vi "SNR_SINAD_THD.vi"(8 "error in (no error)":errorcluster caption="错误输入（无错误）", 9 "THD Power Spectrum":cluster{"f0":dbl, "df":dbl, "magnitude":dbl[]}[](array[cluster]), 10 "Harmonics Data Out":dbl[](array[numeric]), 11 "F_Waveform输入":waveform(dbl) caption="F_Waveform输出") -> (0 "error out":errorcluster caption="错误输出", 1 "THD (dB)":dbl, 2 "SNR Power Spectrum":cluster{"f0":dbl, "df":dbl, "magnitude":dbl[]}[](array[cluster]), 3 "SINAD Power Spectrum":cluster{"f0":dbl, "df":dbl, "magnitude":dbl[]}[](array[cluster]), 4 "SINAD (dB)":dbl, 5 "SNR (dB)":dbl)   [LabVIEW 2019]
uses:
  <vilib>/measure/maspectr.llb/FFT Power Spectrum for 1 Chan.vi
  <vilib>/measure/NI_MAPro.lvlib
  <vilib>/Analysis/NI_AALBase.lvlib
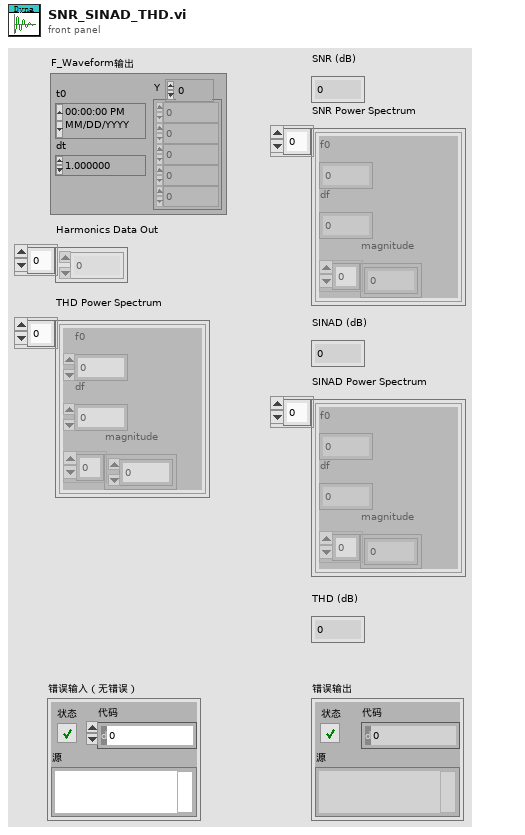
[diagram p1: front panel]
types:
  T1 = enum16{"None ", "Hanning", "Hamming", "Blackman-Harris", "Exact Blackman", "Blackman", "Flat Top", "4 Term B-Harris ", "7 Term B-Harris", "Low Sidelobe"}
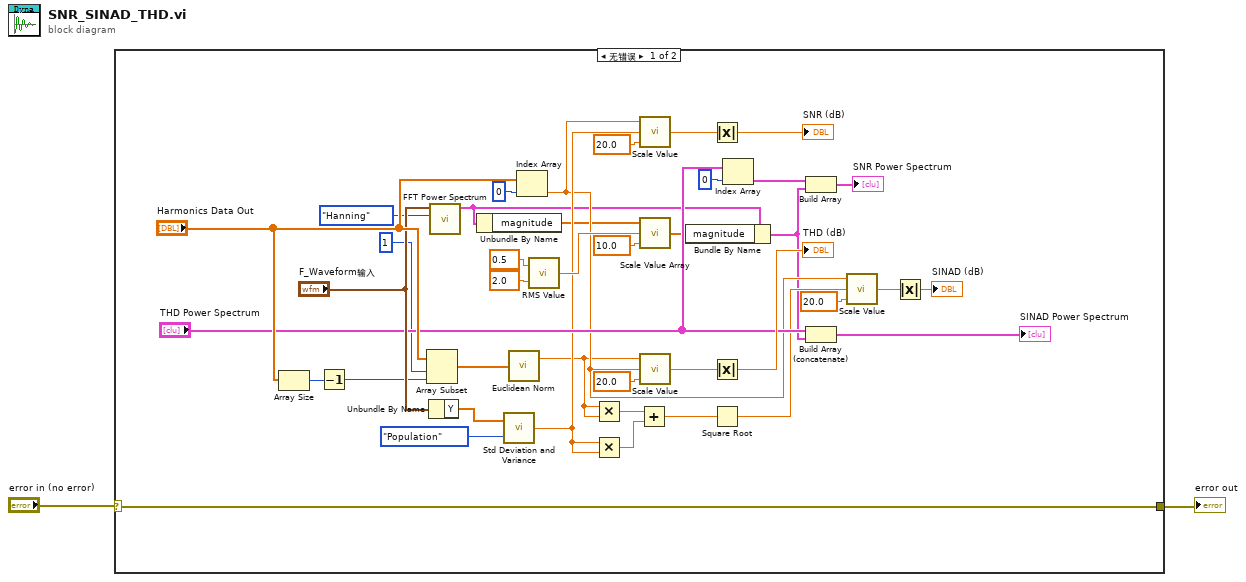
[diagram p0: block diagram]
diagram:
  n1 = case shown="无错误" "error in (no error)" {
    selector: "error in (no error)" -> [w3 w43]
    tunnel: [w3 w43] -> w1
    frame No Error {
      n2 = Array Size(array="Harmonics Data Out") -> (size(s)=w14:i32)
      n3 = Decrement(x=w14) -> (x-1=w13:i32)
      n4 = Array Subset(array="Harmonics Data Out", index=1, length=w13) -> (w10:dbl[])
      n5 = Unbundle By Name("F_Waveform输入") -> ("Y"=w5:dbl[])
      n6 = call-poly <vilib>:"FFT Power Spectrum.vi"("window"=T1."Hanning", "time signal"="F_Waveform输入") -> ("power spectrum"=w23:cluster{"f0":dbl, "df":dbl, "magnitude":dbl[]})  [unwired: 6 in, 3 out]
      n7 = Unbundle By Name(w23) -> ("magnitude"=w20:dbl[])
      n8 = call <vilib>:"Std Deviation and Variance.vi"("X"=w5, "Weighting (Sample)"=enum16{"Sample", "Population"}."Population") -> ("standard deviation"=w29:dbl)  [unwired: 2 out]
      n9 = call <vilib>:"Euclidean Norm.vi"("X"=w10) -> ("root square value"=w24:dbl)  [unwired: 1 out]
      n10 = Index Array(array="Harmonics Data Out", index=0) -> (element=w28:dbl)
      n11 = call "RMS Value.vi"("y"=2.0, "y 2"=0.5 ("y")) -> ("Numeric"=w34:dbl)
      n12 = Multiply(x=w24, y=w24) -> (x*y=w9:dbl)
      n13 = Multiply(x=w29, y=w29) -> (x*y=w8:dbl)
      n14 = Add(x=w9, y=w8) -> (x+y=w7:dbl)
      n15 = call "Scale Value.vi"("y"=20.0, "Numeric"=w29, "root square value"=w28) -> ("THD (dB)"=w31:dbl)
      n16 = call "Scale Value Array.vi"("y"=10.0, "Numeric"=w34, "magnitude 2"=w20) -> ("magnitude"=w21:dbl[])
      n17 = call "Scale Value.vi"("y"=20.0, "Numeric"=w28, "root square value"=w24) -> ("THD (dB)"=w11:dbl)
      n18 = Bundle By Name(cluster=w23, "magnitude"=w21) -> (w16:cluster{"f0":dbl, "df":dbl, "magnitude":dbl[]})
      n19 = Absolute Value(x=w31) -> (abs(x)=→"SNR (dB)":dbl)
      n20 = Absolute Value(x=w11) -> (abs(x)=→"THD (dB)":dbl)
      n21 = Square Root(x=w7) -> (sqrt(x)=w25:dbl)
      n22 = Index Array(array="THD Power Spectrum", index=0) -> (element=w17:cluster{"f0":dbl, "df":dbl, "magnitude":dbl[]})
      n23 = Build Array(w17, w16) -> (→"SNR Power Spectrum":cluster{"f0":dbl, "df":dbl, "magnitude":dbl[]}[])
      n24 = Build Array (concatenate)("THD Power Spectrum", w16) -> (→"SINAD Power Spectrum":cluster{"f0":dbl, "df":dbl, "magnitude":dbl[]}[])
      n25 = call "Scale Value.vi"("y"=20.0, "Numeric"=w25, "root square value"=w28) -> ("THD (dB)"=w27:dbl)
      n26 = Absolute Value(x=w27) -> (abs(x)=→"SINAD (dB)":dbl)
    }
    frame Error {
    }
  }
  "error out" <- w1
